vi "Write.vi"(8 "error in":errorcluster, 10 "Write":T1={"Data (dec)"=0, FALSE, "Index"="``", "Sub-Index"="\u0000", "Data-Size (in Byte)"=1} {"Data-Size (in Byte)" min=1 max=4 step=1 format="%x"; "Data (dec)" step=1}, 11 "ComPort In":refnum<visa-resource-name>="COM1") -> (0 "error out":errorcluster, 3 "ComPort Out":refnum<visa-resource-name>)   [LabVIEW 2021]
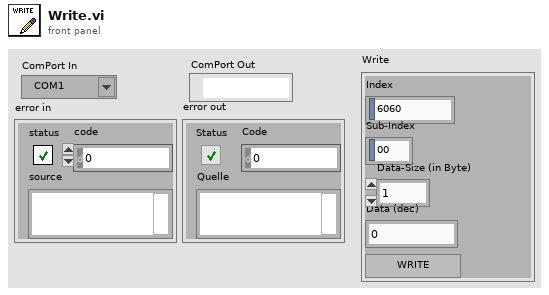
[diagram p1: front panel]
types:
  T1 = cluster{"Data (dec)":i32, bool, "Index":string, "Sub-Index":string, "Data-Size (in Byte)":u8}
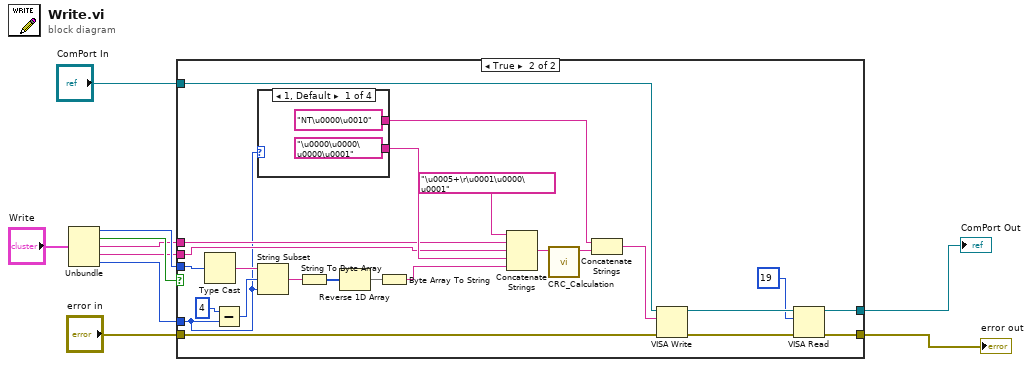
[diagram p0: block diagram]
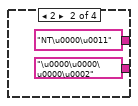
[diagram p3: hidden frame]
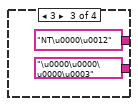
[diagram p4: hidden frame]
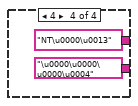
[diagram p5: hidden frame]
diagram:
  n1 = Unbundle("Write") -> ("Data (dec)"=w4:i32, w5:bool, "Index"=w2:string, "Sub-Index"=w1:string, "Data-Size (in Byte)"=w3:u8)
  n2 = case shown="True" w5 {
    tunnel: "ComPort In" -> [w12 w30]
    tunnel: "error in" -> [w11 w29]
    tunnel: [w12 w23] -> w10
    tunnel: [w11 w22] -> w9
    tunnel: w3 -> [_ w16]
    tunnel: w2 -> [_ w21]
    tunnel: w1 -> [_ w20]
    tunnel: w4 -> [_ w13]
    frame False {
    }
    frame True {
      n3 = Type Cast(x=w13) -> (*(type *) &x=w19:string)  [unwired: 1 in]
      n4 = Subtract(x=u8 4, y=w16) -> (x-y=w18:u8)
      n5 = case shown="1, Default" w16 {
        tunnel: ["NT\u0000\u0010" ("Hexadecimal Input String 4") "NT\u0000\u0011" ("Hexadecimal Input String 4") "NT\u0000\u0012" ("Hexadecimal Input String 4") "NT\u0000\u0013" ("Hexadecimal Input String 4")] -> w33
        tunnel: ["\u0000\u0000\u0000\u0001" ("Hexadecimal Input String 4") "\u0000\u0000\u0000\u0002" ("Hexadecimal Input String 4") "\u0000\u0000\u0000\u0003" ("Hexadecimal Input String 4") "\u0000\u0000\u0000\u0004" ("Hexadecimal Input String 4")] -> w36
        frame 1, Default {
        }
        frame 2 {
        }
        frame 3 {
        }
        frame 4 {
        }
      }
      n6 = String Subset(string=w19, offset (0)=w18, length (rest)=w16) -> (substring=w15:string)
      n7 = String To Byte Array(string=w15) -> (unsigned byte array=w26:u8[])
      n8 = Reverse 1D Array(array=w26) -> (reversed array=w28:u8[])
      n9 = Byte Array To String(unsigned byte array=w28) -> (string=w31:string)
      n10 = Concatenate Strings("\u0005+\r\u0001\u0000\u0001" ("Hexadecimal Input String 4"), w21, w20, w36, w31) -> (w25:string)
      n11 = call "CRC_Calculation.vi"("CMD"=w25) -> ("CMD + CRC"=w24:string)  [unwired: 10 in]
      n12 = Concatenate Strings(w33, w24) -> (w14:string)
      n13 = VISA Write(VISA resource name=w30, write buffer=w14, error in (no error)=w29) -> (VISA resource name out=w34:refnum<visa-resource-name>, error out=w35:errorcluster)  [unwired: 1 out]
      n14 = VISA Read(VISA resource name=w34, byte count=u32 19, error in (no error)=w35) -> (VISA resource name out=w23:refnum<visa-resource-name>, error out=w22:errorcluster)  [unwired: 2 out]
    }
  }
  "ComPort Out" <- w10
  "error out" <- w9
